vi "TDMS Advanced - Basic Asynchronously.vi"() -> ()   [LabVIEW 2020]
panel:
  out "Waveform Graph":u32[](graph)
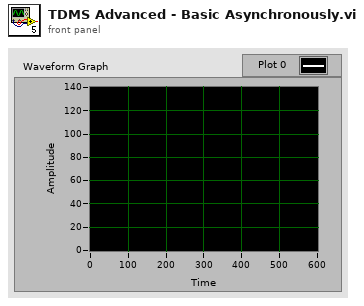
[diagram p1: front panel]
types:
  T1 = enum16{"open", "open or create", "create or replace", "create", "open (read-only)"}
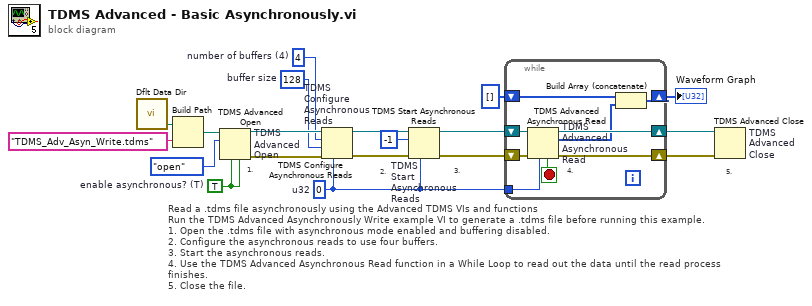
[diagram p0: block diagram]
diagram:
  w5 = u32 0  # u32
  w11 = u32 128  # buffer size
  w12 = u32 4  # number of buffers (4)
  w15 = TRUE  # enable asynchronous? (T)
  # "3."
  # "2."
  # "Read a .tdms file asynchronously using the Advanced TDMS VIs and functions\nRun the TDMS Advanced Asynchronously Write example VI to generate a .tdms file before running this example.\n1. Open the .tdms file with asynchronous mode enabled and buffering disabled.\n2. Configure the asynchronous reads to use four buffers.\n3. Start the asynchronous reads.\n4. Use the TDMS Advanced Asynchronous Read function in a While Loop to read out the data until the read process finishes.\n5. Close the file."
  # "1."
  # "5."
  n1 = call <vilib>:"Dflt Data Dir.vi"() -> ("App:Default Data Directory"=w16:path)
  n2 = Build Path(base path=w16, name or relative path="TDMS_Adv_Asyn_Write.tdms") -> (appended path=w18:path)
  n3 = TDMS Advanced Open "TDMS\nAdvanced\nOpen"(4:w15, 6:w15, 10:T1."open" ("operation (0:open)"), 11:w18) -> (0:w13:errorcluster, 3:w14:refnum<k34>)  [unwired: 1 in, 1 out]
  n4 = TDMS Configure Asynchronous Reads "TDMS\nConfigure\nAsynchronous\nReads"(6:w5, 8:w13, 9:w11, 10:w12, 11:w14) -> (0:w9:errorcluster, 3:w10:refnum<k34>)  [unwired: 1 in]
  n5 = TDMS Start Asynchronous Reads "TDMS\nStart\nAsynchronous\nReads"(6:w5, 8:w9, 10:i64 -1 ("total count (-1)"), 11:w10) -> (0:w6:errorcluster, 3:w7:refnum<k34>)
  n6 = while {
    shift-right: [w25] -> w3
    shift-left: w7 -> [w28]
    shift-right: [w26] -> w4
    shift-left: w6 -> [w27]
    tunnel: w5 -> [w24]
    shift-right: [w20] -> w1
    shift-left: u32[] [] ("data") -> [w22]
    stop <- w23 stop-if-true
    # "4."
    n7 = TDMS Advanced Asynchronous Read "TDMS\nAdvanced\nAsynchronous\nRead"(6:w24, 8:w27, 11:w28) -> (0:w26:errorcluster, 2:w21:u32[], 3:w25:refnum<k34>, 4:w23:bool)
    n8 = Build Array (concatenate)(w22, w21) -> (w20:u32[])
  }
  "Waveform Graph" <- w1
  n9 = TDMS Advanced Close "TDMS\nAdvanced\nClose"(8:w4, 11:w3) -> ()  [unwired: 2 in, 2 out]
